vi "parseImageData.vi"(8 "error in (no error)":errorcluster, 11 "results-JSON string":string) -> (0 "error out":errorcluster, 2 "meta data":T1[][](array[typedef]), 3 "xyData":dbl[][][][](array[numeric]))   [LabVIEW 2023, in "CCD.lvclass"]
doc: "Helper VI to parse the ccd data to a LV 2D image array."
uses:
  CCD.lvclass
  CCDImageData.ctl
  81c9510d-da94-45eb-b341-4ac2c5dcdc17.vi
  <vilib>/JDP Science/JSONtext/Next JSON Value.vi
  <vilib>/JDP Science/JSONtext/String Subset.vi
  <vilib>/JDP Science/JSONtext/Parsing/Advance past next JSON Value (inlined COPY).vi
  <vilib>/JDP Science/JSONtext/Parsing/Advance past whitespace.vi
  <vilib>/JDP Science/JSONtext/Parsing/Advance past String.vi
  <vilib>/JDP Science/JSONtext/Parsing/Advance past Number.vi
  <vilib>/JDP Science/JSONtext/Parsing/Advance past Line Ending.vi
  <vilib>/JDP Science/JSONtext/Parsing/Parse Full Path or Item Name.vi
  <vilib>/JDP Science/JSONtext/Parsing/Advance past Array.vi
  <vilib>/JDP Science/JSONtext/Parsing/Advance past Object.vi
  <vilib>/JDP Science/JSONtext/support/Error Cluster From Code.vi
  <vilib>/JDP Science/JSONtext/Offset/Find Item Locations by Path.vi
  <vilib>/JDP Science/JSONtext/JSON text to Variant.vi
  <vilib>/JDP Science/JSONtext/LVClass Serializer/JSONtext LVClass Serializer.lvclass
  <vilib>/JDP Science/JSONtext/JSONtext.lvlib
panel:
  # "acquisition"
  # "ROI"
  # "pixel-number (=wavelength)"
  # "choose: pixel position - intensity"
  # "Connector Pane"
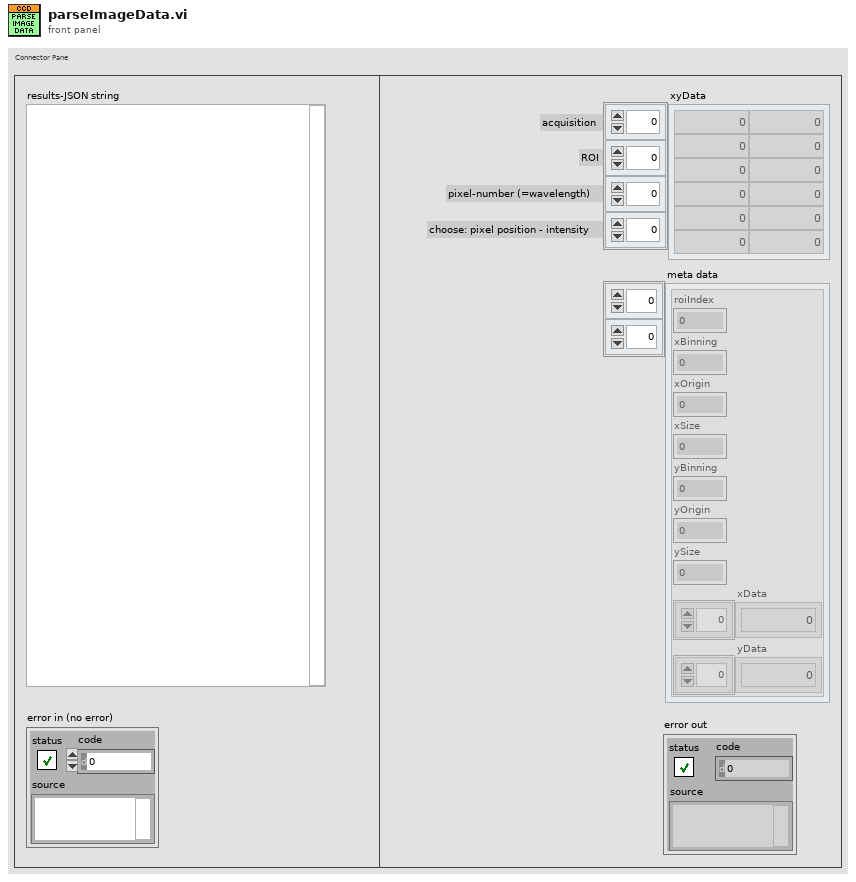
[diagram p1: front panel]
types:
  T1 = typedef "CCD.lvclass/CCDImageData.ctl" = cluster{"roiIndex":i32, "xBinning":i32, "xOrigin":i32, "xSize":i32, "yBinning":i32, "yOrigin":i32, "ySize":i32, "xData":dbl[], "yData":dbl[]}
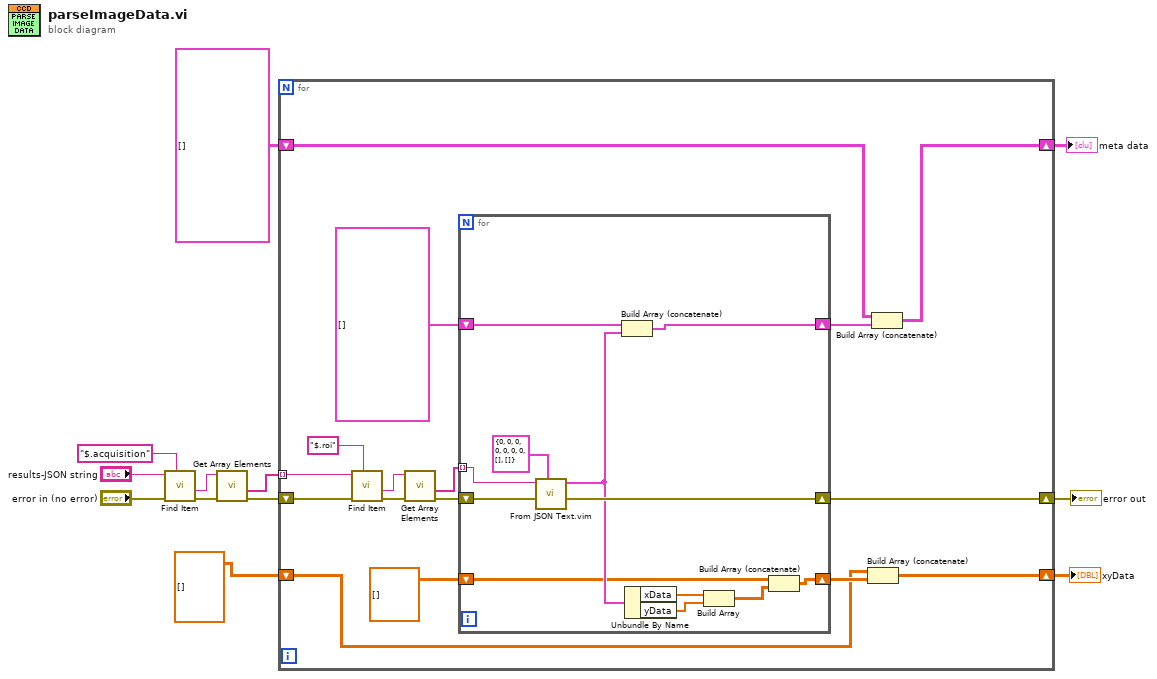
[diagram p0: block diagram]
diagram:
  n1 = call <vilib>:"Find Item.vi"("$Path or Item Name"="$.acquisition", "error in (no error)"="error in (no error)", "JSON"="results-JSON string") -> ("error out"=w9:errorcluster, "<JSON>"=w8:string)  [unwired: 5 in, 2 out]
  n2 = call <vilib>:"Get Array Elements.vi"("error in (no error)"=w9, "JSON"=w8) -> ("error out"=w12:errorcluster, "<JSON>"=w11:string[])  [unwired: 7 in, 1 out]
  n3 = for {
    tunnel: w11 -> [w22] mode=indexing
    shift-right: [w23] -> w7
    shift-left: w12 -> [w25]
    shift-right: [w19] -> w4
    shift-left: T1[][] [] -> [w20]
    shift-right: [w16] -> w2
    shift-left: dbl[][][][] [] -> [w15]
    n4 = call <vilib>:"Find Item.vi"("$Path or Item Name"="$.roi", "error in (no error)"=w25, "JSON"=w22) -> ("error out"=w27:errorcluster, "<JSON>"=w26:string)  [unwired: 5 in, 2 out]
    n5 = call <vilib>:"Get Array Elements.vi"("error in (no error)"=w27, "JSON"=w26) -> ("error out"=w24:errorcluster, "<JSON>"=w21:string[])  [unwired: 7 in, 1 out]
    n6 = for {
      shift-right: [w37] -> w23
      shift-left: w24 -> [w38]
      tunnel: w21 -> [w36] mode=indexing
      shift-right: [w40] -> w13
      shift-left: T1[] [] -> [w39]
      shift-right: [w33] -> w17
      shift-left: dbl[][][] [] -> [w34]
      n7 = call "From JSON Text.vim"("Data Type and Default Value"=T1 {"roiIndex"=0, "xBinning"=0, "xOrigin"=0, "xSize"=0, "yBinning"=0, "yOrigin"=0, "ySize"=0, "xData"=[], "yData"=[]} ("Gain"), "error in (no error)"=w38, "JSON"=w36) -> ("error out"=w37:errorcluster, "Data out"=w35:T1)  [unwired: 7 in]
      n8 = Build Array (concatenate)(w39, w35) -> (w40:T1[])
      n9 = Unbundle By Name(w35) -> ("xData"=w30:dbl[], "yData"=w31:dbl[])
      n10 = Build Array(w30, w31) -> (w29:dbl[][])
      n11 = Build Array (concatenate)(w34, w29) -> (w33:dbl[][][])
    }
    n12 = Build Array (concatenate)(w15, w17) -> (w16:dbl[][][][])
    n13 = Build Array (concatenate)(w20, w13) -> (w19:T1[][])
  }
  "error out" <- w7
  "xyData" <- w2
  "meta data" <- w4
